vi "ConfigFileParser.vi"(0 "Path":path, 11 "error in":errorcluster) -> (3 "Configuration":string[][](array[string]), 4 "General Settings":string[][](array[string]), 6 "Program":string[][](array[string]), 8 "Loop Microscope Settings":string[][](array[string]), 10 "Positions":string[][](array[string]), 15 "error out":errorcluster)   [LabVIEW 2018, in "Config.lvlib"]
uses:
  Config.lvlib
  <vilib>/xml/Load XML File.vi
  <vilib>/xml/NI_XML.lvlib
  <resource>/objmgr/DOMUserDefRef.rc
panel:
  out "XML":string
  out "Parse Errors":string
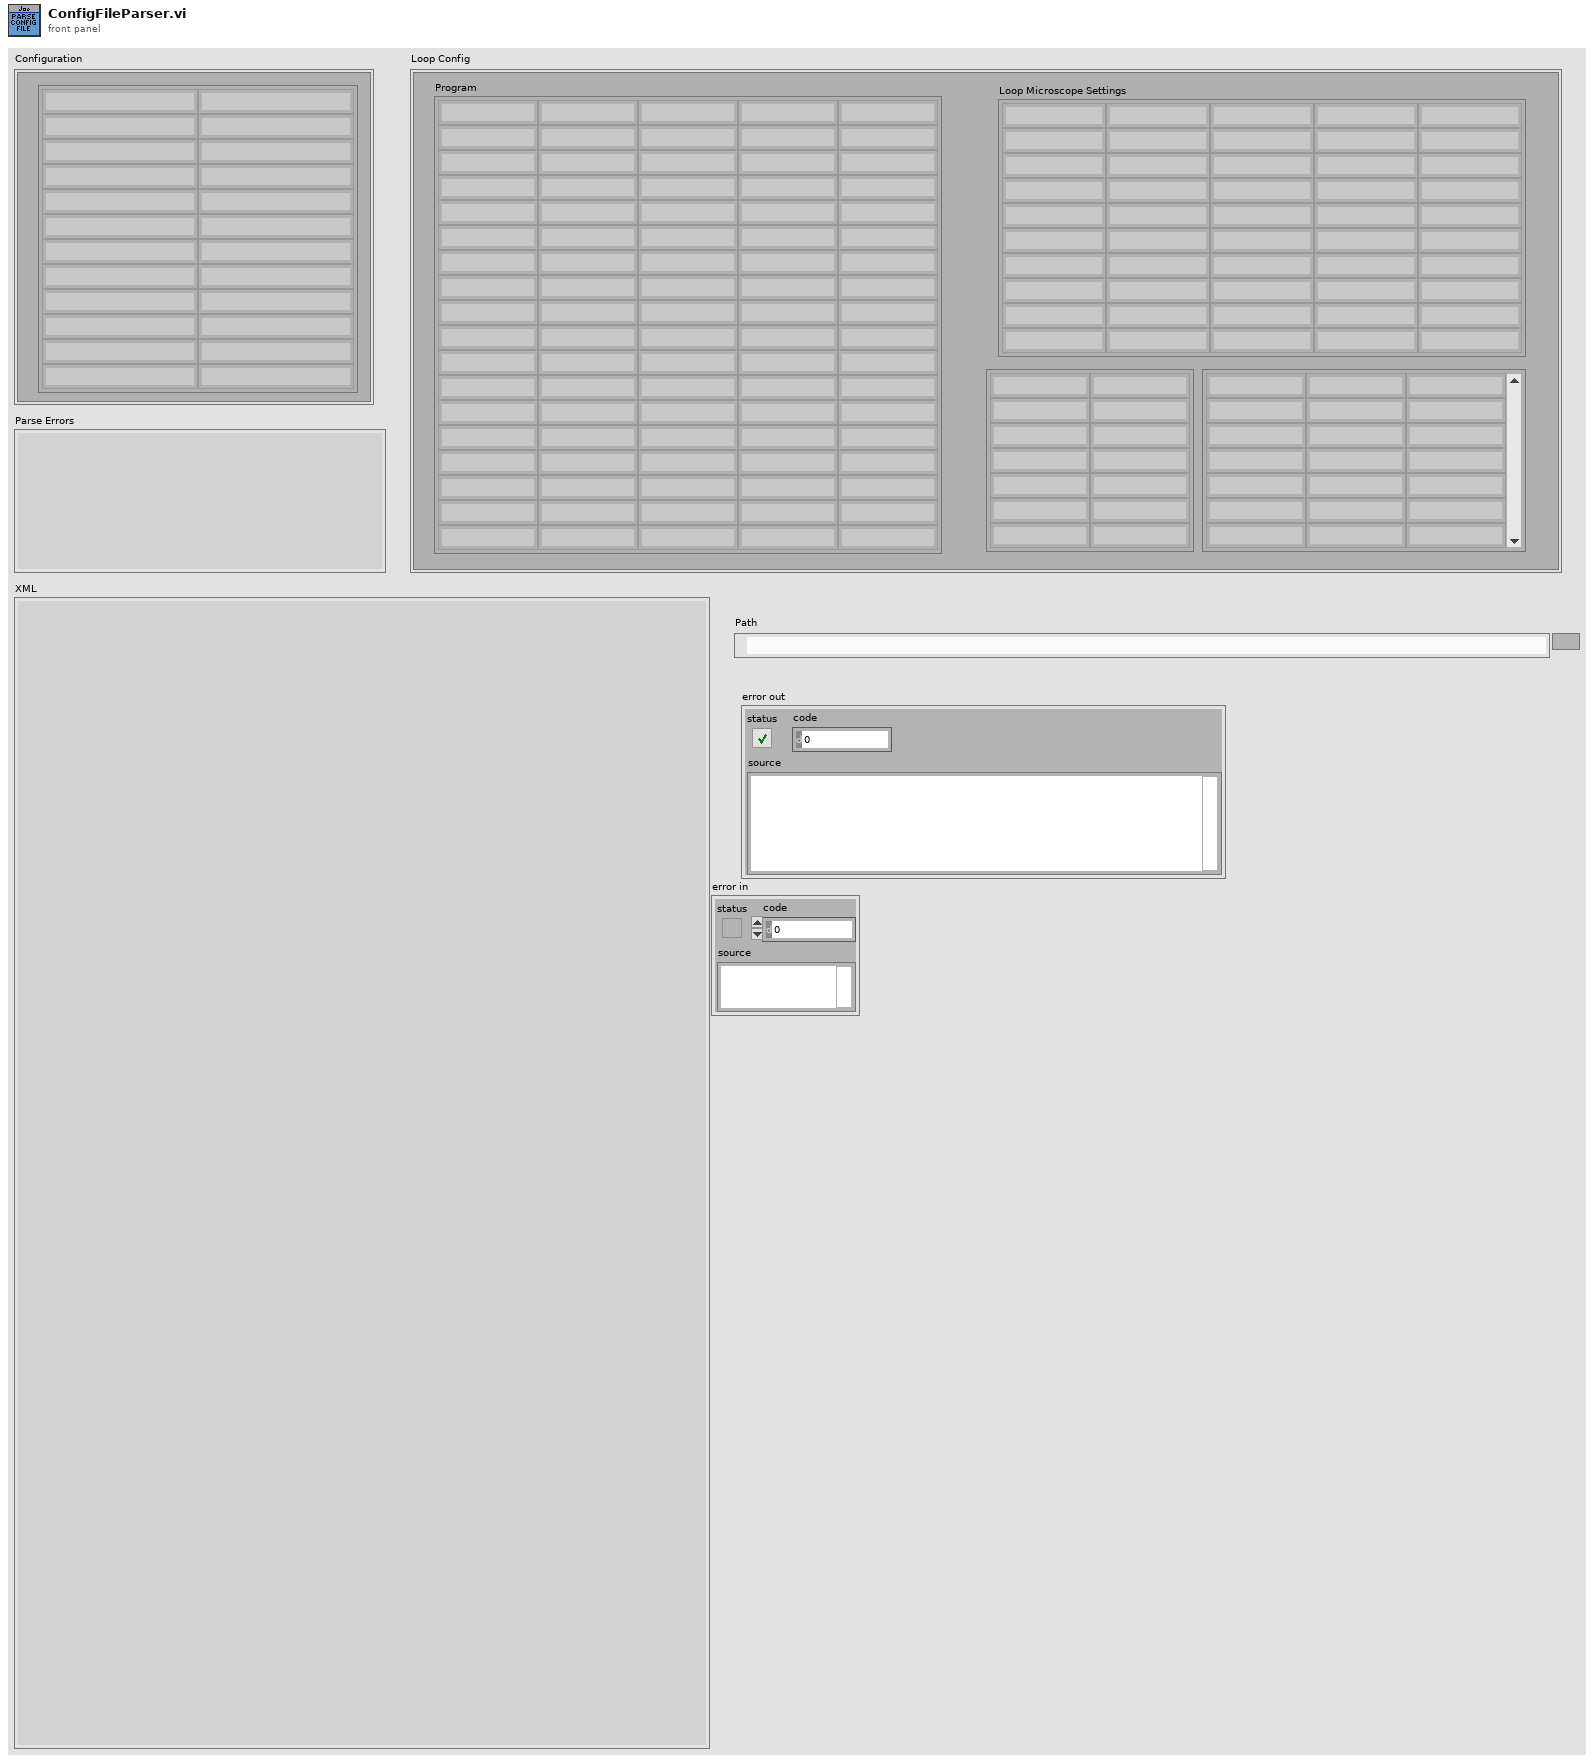
[diagram p1: front panel]
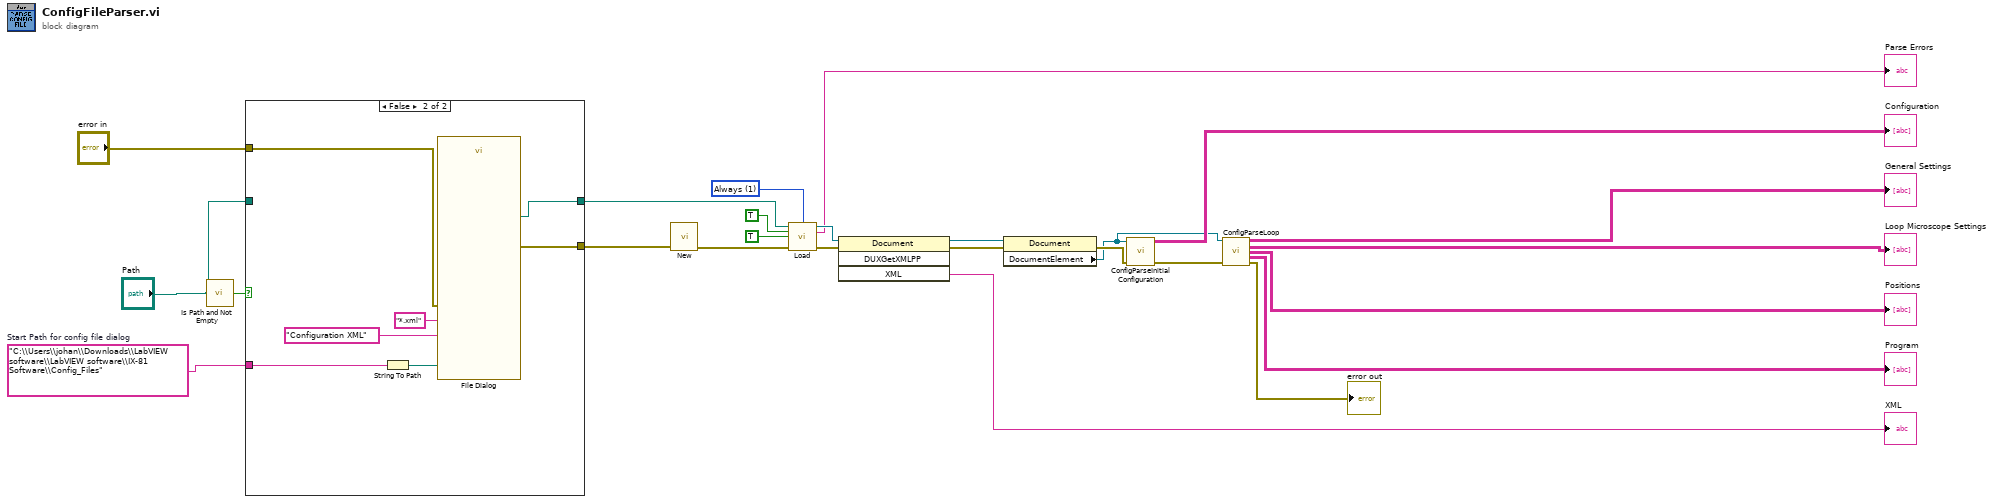
[diagram p0: block diagram]
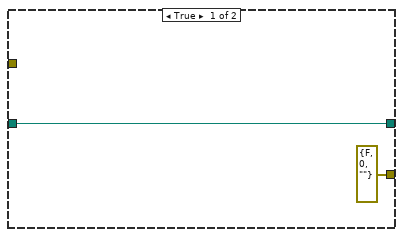
[diagram p2: hidden frame]
diagram:
  w2 = "C:\\Users\\johan\\Downloads\\LabVIEW software\\LabVIEW software\\IX-81 Software\\Config_Files"  # Start Path for config file dialog
  w19 = 1 items=["Never", "Always", "Auto"] ("validate on load (Auto)")
  n1 = call <vilib>:"Is Path and Not Empty.vi"("path"="Path") -> ("Is Path and Not Empty?"=w8:bool)  [unwired: 4 in]
  n2 = case shown="False" w8 {
    tunnel: [w27 w32] -> w15
    tunnel: [errorcluster {"status"=FALSE, "code"=0, "source"=""} ("error out") w31] -> w14
    tunnel: "Path" -> [w27 _]
    tunnel: w2 -> [_ w30]
    tunnel: "error in" -> [_ w28]
    frame True {
    }
    frame False, Default {
      n3 = String To Path(string=w30) -> (path=w29:path)
      n4 = call "File Dialog"("start path"=w29, "error in"=w28, "pattern (all files)"="*.xml", "pattern label"="Configuration XML") -> ("selected path"=w32:path, "error out"=w31:errorcluster)  [unwired: 8 in, 2 out]
    }
  }
  n5 = call <vilib>:"New.vi"("error in (no error)"=w14) -> ("error out"=w24:errorcluster)  [unwired: 7 in, 1 out]
  n6 = call-poly <vilib>:"Load.vi"("path to XML document"=w15, "validate on load (Auto)"=w19, "process namespaces (False)"=TRUE, "process schema (False)"=TRUE, "error in (no error)"=w24) -> ("DOM document out"=w22:refnum<k20>, "parse errors"=→"Parse Errors":string, "error out"=w21:errorcluster)  [unwired: 8 in]
  n7 = invoke class="Document" method="DUXGetXMLPP"(reference=w22, error in=w21) -> (reference out=w17:refnum<k20>, error out=w16:errorcluster, "XML"=→"XML":string)  [unwired: 2 in, 1 out]
  n8 = property class="Document"(reference=w17, error in=w16) -> (error out=w6:errorcluster, "DocumentElement"=w5:refnum<k20>)  [unwired: 1 out]
  n9 = call "ConfigParseInitialConfiguration.vi"("error in (no error)"=w6, "Root Refnum in"=w5) -> ("error out"=w4:errorcluster, "Configuration Array"=→"Configuration":string[][])  [unwired: 8 in]
  n10 = call "ConfigParseLoop.vi"("Root Refnum in"=w5, "error in (no error)"=w4) -> ("General Settings"=→"General Settings":string[][], "Loop Microscope Settings"=→"Loop Microscope Settings":string[][], "Position Settings"=→"Positions":string[][], "Program"=→"Program":string[][], "error out"=→"error out":errorcluster)  [unwired: 9 in]
